vi "Update Servo Filter.vi"(4 "error in (no error)":errorcluster, 6 "Axis (0)":i32 min=0 max=3, 7 "VISA resource name":refnum<visa-resource-name>) -> (0 "error out":errorcluster, 3 "VISA resource name out":refnum<visa-resource-name>)   [LabVIEW 2012, in "Newport ESP301.lvlib"]
doc: "This command is used to make active the latest entered PID parameters. Any new value for Kp, Ki, Kd and maximum following error are not being used in the PID loop calculation until UF command is received. This assures that the parameters are loaded simultaneously, without any transitional glitches in the loop.\n\nIf the axis specifier <B>Axis (0)</B> is missing or set to 0 , the controller updates the filters for all axes. If <B>Axis (0)</B> is a number between 1 and 3, the controller updates only the filter for the specified axis."
uses:
  Newport ESP301.lvlib
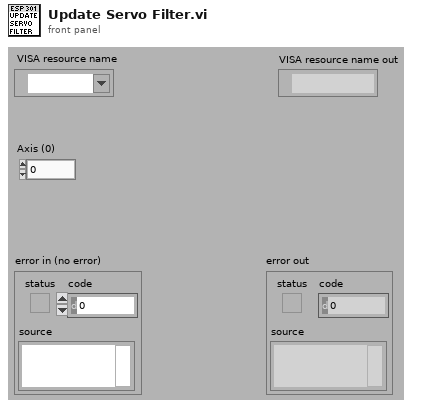
[diagram p1: front panel]
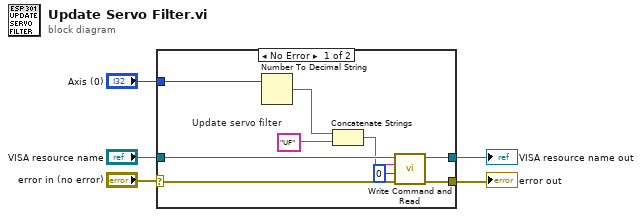
[diagram p0: block diagram]
diagram:
  n1 = case shown="No Error" "error in (no error)" {
    selector: "error in (no error)" -> [w11 w16]
    tunnel: [w13 w16] -> w5
    tunnel: "VISA resource name" -> [w14 w15]
    tunnel: [w12 w15] -> w4
    tunnel: "Axis (0)" -> [w8 _]
    frame No Error {
      w9 = "UF"  # Update servo filter
      n2 = Number To Decimal String(number=w8) -> (decimal integer string=w7:string)  [unwired: 1 in]
      n3 = Concatenate Strings(w7, w9) -> (w6:string)
      n4 = call "Write Command and Read.vi"("error in (no error)"=w11, "Bytes to read (100)"=u32 0, "Command"=w6, "VISA resource name"=w14) -> ("error out"=w13:errorcluster, "VISA resource name out"=w12:refnum<visa-resource-name>)  [unwired: 1 in, 3 out]
    }
    frame Error {
    }
  }
  "error out" <- w5
  "VISA resource name out" <- w4
